vi "bofxy backup.vi"(10 "Y":dbl[](array[numeric]) format="%#_13g", 11 "X":dbl[](array[numeric]) format="%#_13g") -> (1 "dB dy":T1, 2 "dB dx":T2, 3 "B":cluster{"Bx":dbl[], "By":dbl[], "Bz":dbl[]})   [LabVIEW 2017]
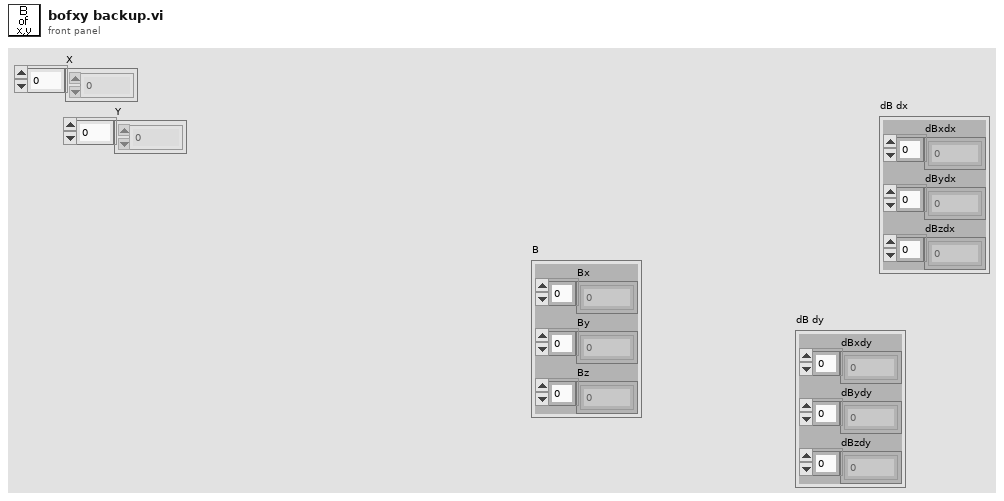
[diagram p1: front panel]
types:
  T1 = cluster{"dBxdy":dbl[], "dBydy":dbl[], "dBzdy":dbl[]}
  T2 = cluster{"dBxdx":dbl[], "dBydx":dbl[], "dBzdx":dbl[]}
  T3 = cluster{"dBydx":dbl[], "dBxdx":dbl[], "dBzdx":dbl[]}
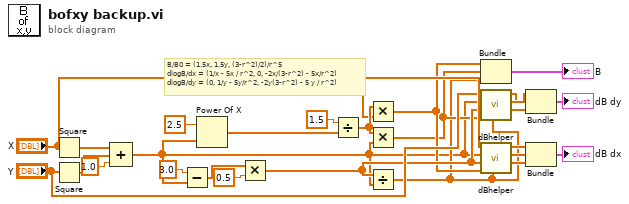
[diagram p0: block diagram]
diagram:
  # "B/B0 = (1.5x, 1.5y, (3-r^2)/2)/r^5\ndlogB/dx = (1/x - 5x / r^2, 0, -2x/(3-r^2) - 5x/r^2)\ndlogB/dy = (0, 1/y - 5y/r^2, -2y(3-r^2) - 5 y / r^2)"
  n1 = Square(x="X") -> (x^2=w26:dbl[])
  n2 = Square(x="Y") -> (x^2=w17:dbl[])
  n3 = Compound Arithmetic op=ADD(w26, w17, 1.0) -> (w1:dbl[])
  n4 = Subtract(x=3.0, y=w1) -> (x-y=w19:dbl[])
  n5 = Power Of X(1:w1, 2:2.5) -> (0:w22:dbl[])
  n6 = Multiply(x=w19, y=0.5) -> (x*y=w14:dbl[])
  n7 = Divide(x=1.5, y=w22) -> (x/y=w21:dbl[])
  n8 = Multiply(x=w21, y="X") -> (x*y=w4:dbl[])
  n9 = Multiply(x=w21, y=w1) -> (x*y=w3:dbl[])
  n10 = Divide(x=w14, y=w1) -> (x/y=w2:dbl[])
  n11 = Bundle(w4, w3, w2) -> (→"B":cluster{dbl[], dbl[], dbl[]})  [unwired: 1 in]
  n12 = call "dBhelper.vi"("Bz"=w2, "Bx"=w3, "(3-r^2)/2"=w14, "rsq"=w1, "X"="Y") -> ("dBzdx"=w8:dbl[], "dBydx"=w10:dbl[], "dBxdx"=w9:dbl[])  [unwired: 4 in]
  n13 = call "dBhelper.vi"("Bz"=w2, "Bx"=w4, "(3-r^2)/2"=w14, "rsq"=w1, "X"="X") -> ("dBzdx"=w11:dbl[], "dBydx"=w12:dbl[], "dBxdx"=w13:dbl[])  [unwired: 4 in]
  n14 = Bundle("dBydx"=w10, "dBxdx"=w9, "dBzdx"=w8) -> (→"dB dy":T3)  [unwired: 1 in]
  n15 = Bundle("dBxdx"=w13, "dBydx"=w12, "dBzdx"=w11) -> (→"dB dx":T2)  [unwired: 1 in]
